vi "Functional Imaging Viewer.vi"(8 "error in (no error)":errorcluster, 11 "Experiment data folder path":path) -> ()   [LabVIEW 2013]
uses:
  Typedefs/ROI selector array-ROI vis.ctl
  xcontrol/Interface VIs/Interface typedefs/Interface-ROI selection cluster.ctl
  Typedefs/ROI ID Enum.ctl
  xcontrol/XGrapher.xctl
  Typedefs/Group sel cluster.ctl
  Typedefs/ROI visibility mode.ctl
  Typedefs/Functional Imging UI Refs.ctl
  Typedefs/Groups array referecne.ctl
  SubVIs/ROI grouping window/Typedefs/ROI grp-process states enum.ctl
  Typedefs/Registered event names enum.ctl
  Globals/gl_Funct imaging UI.vi
  Global variables/gl_Functional Imaging-Global variables.vi
panel:
  out "#of selected groups":i32 caption="MiniScans selected" format="%.0f Miniscans selected"
  out "Index of POI clicked on":i16
  out "Image":T1(plugin-control)
  out "Doc Min":dbl
  out "Doc Max":dbl
  in  "Z-Plane Selector":i32(c297)=7 caption="Z-Plane"
  out "Index of group clicked on":i16
  in  "ROI vis. mode":T2
  in  "Max Z-Projection":bool
  in  "Channel":u16(ring)=1 items=["Red", "Green"]
  in  "Intensity Zoom":cluster{u16, u16}(slide)={0, 694} scale=0.0..4095.0
  in  "Index of miniscan point to visualise":i32=1 min=1 max=61 step=1 format="Point %.0f"
  in  "Waveform selector":u16(ring) items=["Cursor on ROI 1 (MiniScan)"]
  out "XGrapher":T7(xcontrol)
  in  "Deselect all groups":bool=TRUE
  in  "Deselect all ROI":bool=TRUE
  out "Group info":string="0 of 0 groups selected"
  in  "[Groups]":T8[](array[typedef]) caption="Groups"
  out "Miniscan info":string="0 of 0 miniscans selected"
  out "POI info":string="0 of 0 POI selected"
  in  "Trial No.":i32=1 caption="Selected Trial" min=1 max=2 format="Trial %.0f"
  out "Number of Trials (ind1)":u16 min=1 max=16 format="of %.0d"
  in  "Smoothing":i32(slide) scale=0.0..10.0
  out "Number of Trials (ind 2)":u16 caption="Number of trials"
  out "Total # of points":i32 caption="Total number\nof loaded points"
  out "POI data points in each trial":i32
  out "#of selected POI":i32 caption="POI selected" format="%.0f POI selected"
  out "POI available":i32 caption="POI Available" format="%.0f POI available"
  out "MiniScans Available":i32 format="%.0f Miniscans available"
  out "#of selected MiniScans":i32 caption="MiniScans selected" format="%.0f Miniscans selected"
  in  "Defer graph updates":bool caption="Defer graph updates\non cursor move"
  in  "[ROI vis]":T9 caption="ROIs" {"ROI number" min=1 max=4 format="ROI %.0f"}
  in  "Show All":bool
  in  "Normalize":bool
  in  "POI Averaging":bool
  in  "Trial Cursor Enabled":bool caption="Trial Tracking Cursors"
  # "Cursors Settings"
  # "Post Processing Settings"
  # "Information"
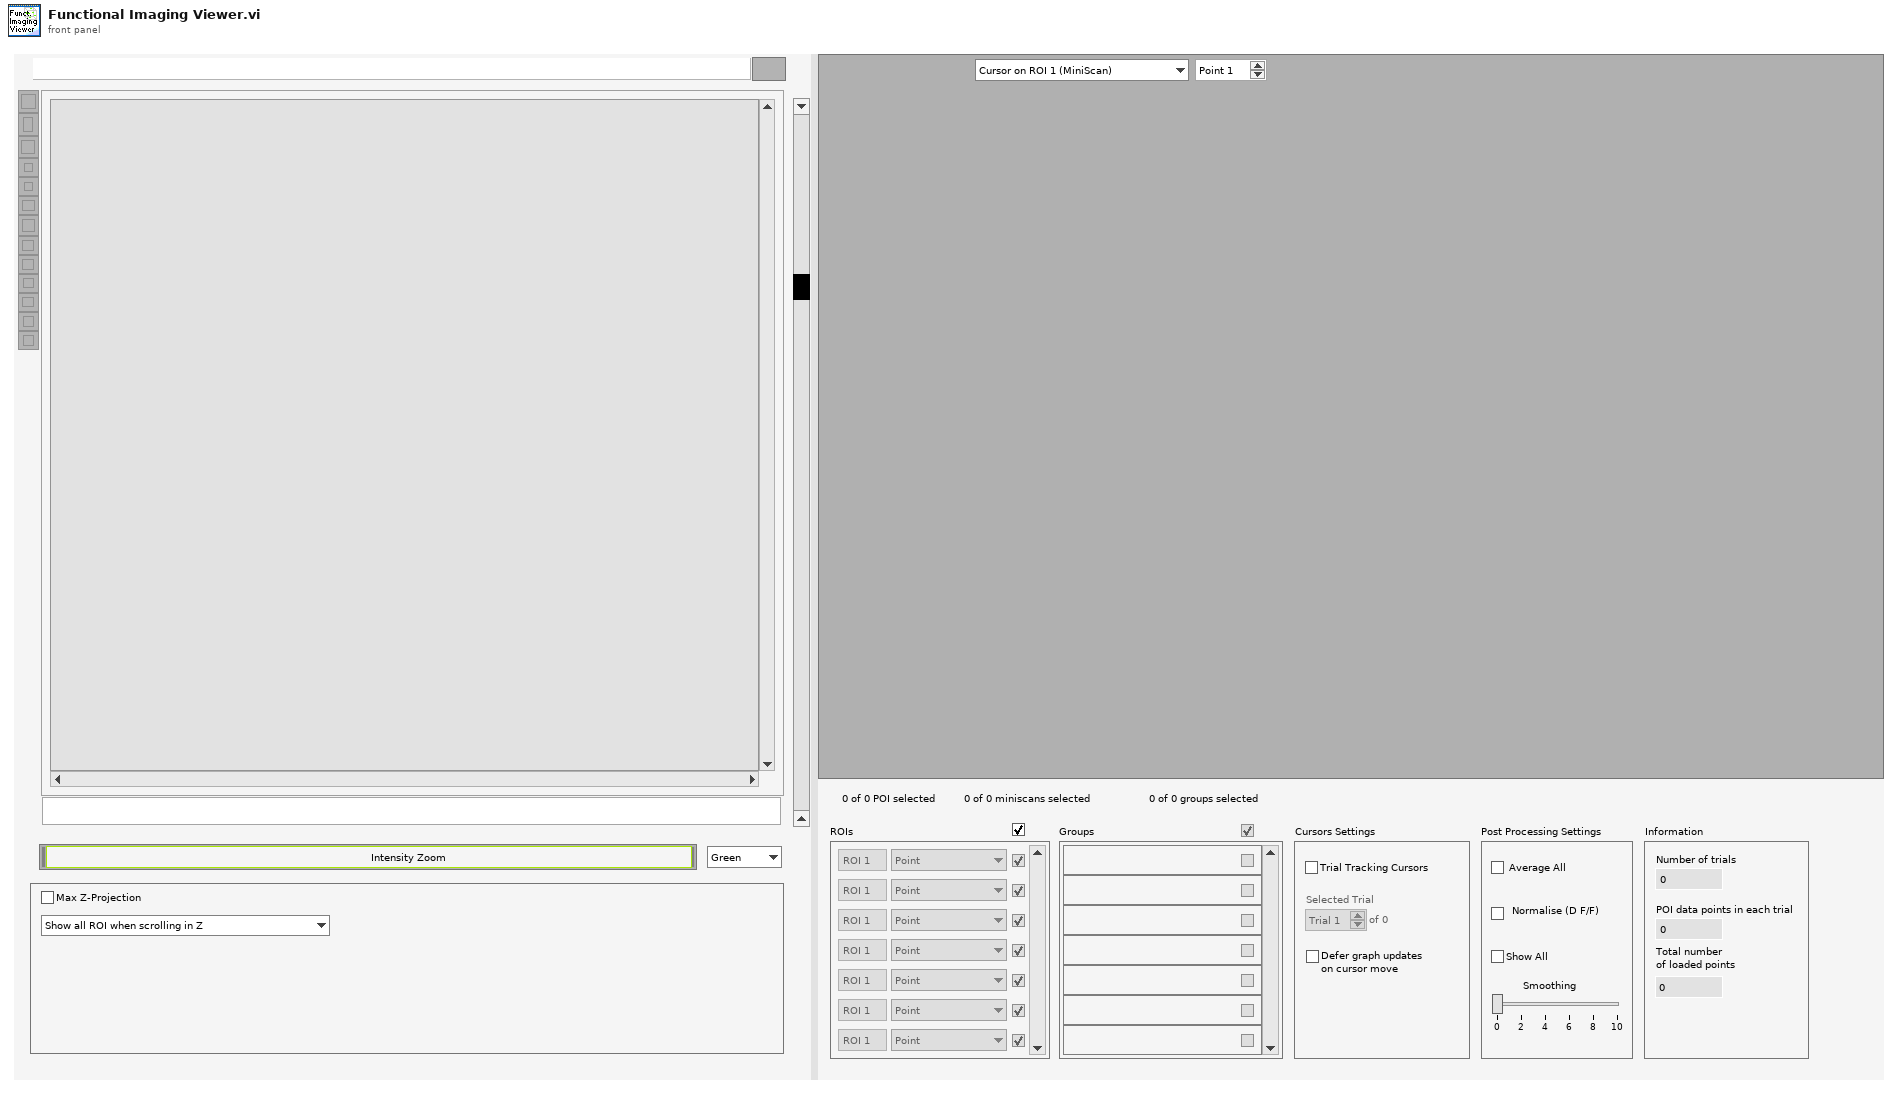
[diagram p1: front panel]
types:
  T1 = typedef "IMAQ Image.ctl" = refnum<image>
  T2 = typedef "ROI visibility mode.ctl" = enum16{"Show all ROI when scrolling in Z", "Show only selected ROI when scrolling in Z"}
  T3 = typedef "Xctrl-Data array.ctl" = T4[]
  T4 = typedef "XGrapher.xctl/Xcrtl-Data format definition.ctl" = cluster{"Plot.Plot Name":string, "Data":T5, "Timeline data":T5, "Type":T6, "Points per cycle":u16, "ROI index":u16}
  T5 = typedef "XGrapher.xctl/Xctl-XY data type definition.ctl" = cluster{"X-Axis values":sgl[], "Y-Axis values (s)":i32[]}
  T6 = typedef "Xctrl-ROI type enum.ctl" = enum16{"POI", "Mini-scan", "Group"}
  T7 = cluster{"Data & info by ROI index":T3, "Index of selected plot":u16, "Points in each trial":i32, "POI Averaging":bool, "Reset graph X-axis scaling":bool, "Selected point index in MSCN (unity based)":u16}
  T8 = typedef "Group sel cluster.ctl" = cluster{"Group number":string, "Group Name":string, "Visibility":bool, "Highlight":bool}
  T9 = typedef "ROI selector array-ROI vis.ctl" = T10[]
  T10 = typedef "Interface-ROI selection cluster.ctl" = cluster{"ROI number":i32, "ROI ID":T11, "Visibility":bool}
  T11 = typedef "ROI ID Enum.ctl" = enum16{"Point", "MiniScan", "Comp. MiniScan", "Rectangle", "Comp. volume", "Arb. plane point"}
  T12 = typedef "Functional Imging UI Refs.ctl" = cluster{"Menu ref":refnum<k9>, "Image control":refnum<vi>, "VI ref":refnum<vi>, "XGrapher":refnum<vi>, "Smoothing":refnum<vi>, "POI Averaging":refnum<vi>, "Normalize":refnum<vi>, "POI data points in each trial":refnum<vi>, "Channel":refnum<vi>, "Experiment data folder path":refnum<vi>, "[ROI vis]":refnum<vi>, "[Groups] visbl":T13, "Group Name":refnum<vi>, "POI index":refnum<vi>, "Trial No.":refnum<vi>, "Intensity Zoom":refnum<vi>, "Trial Cursor Enabled":refnum<vi>, "Number of Trials (ind 1)":refnum<vi>, "Number of Trials (ind 2)":refnum<vi>, "MiniScans Available":refnum<vi>, "POI Available":refnum<vi>, "Defer graph updates":refnum<vi>, "Waveform selector":refnum<vi>, "#of selected POI":refnum<vi>, "#of selected MiniScans":refnum<vi>, "#of selected groups":refnum<vi>, "Max Z-Projection":refnum<vi>, "Z-Plane Selector":refnum<vi>, "Index of miniscan point to visualise":refnum<vi>, "ROI vis. mode":refnum<vi>, "Total # of points":refnum<vi>, "Index of group clicked on":refnum<vi>, "Pane 1":refnum<vi>, "Pane 2":refnum<vi>, "Pane 3":refnum<vi>, "Pane 4":refnum<vi>, "Pane 5":refnum<vi>, "Pane 6":refnum<vi>, "Deselect all ROI":refnum<vi>, "Deselect all groups":refnum<vi>}
  T13 = typedef "Groups array referecne.ctl" = refnum<vi>
  T14 = typedef "Registered event names enum.ctl" = enum16{"Register", "Load dataset in funct viewer", "Re-process data", "Export selected ROI data-full"}
  T15 = typedef "ROI grp-process states enum.ctl" = enum16{"Open window", "Stop loop"}
  T16 = typedef "FuncImg-Events registration ref.ctl" = refnum<event-registration>
  T17 = typedef "eventsource.ctl" = u32
  T18 = typedef "Interface-ROI type enum.ctl" = enum16{"POI", "Mini-scan"}
  T19 = typedef "LVPoint32TypeDef.ctl" = cluster{"Horizontal":i32, "Vertical":i32}
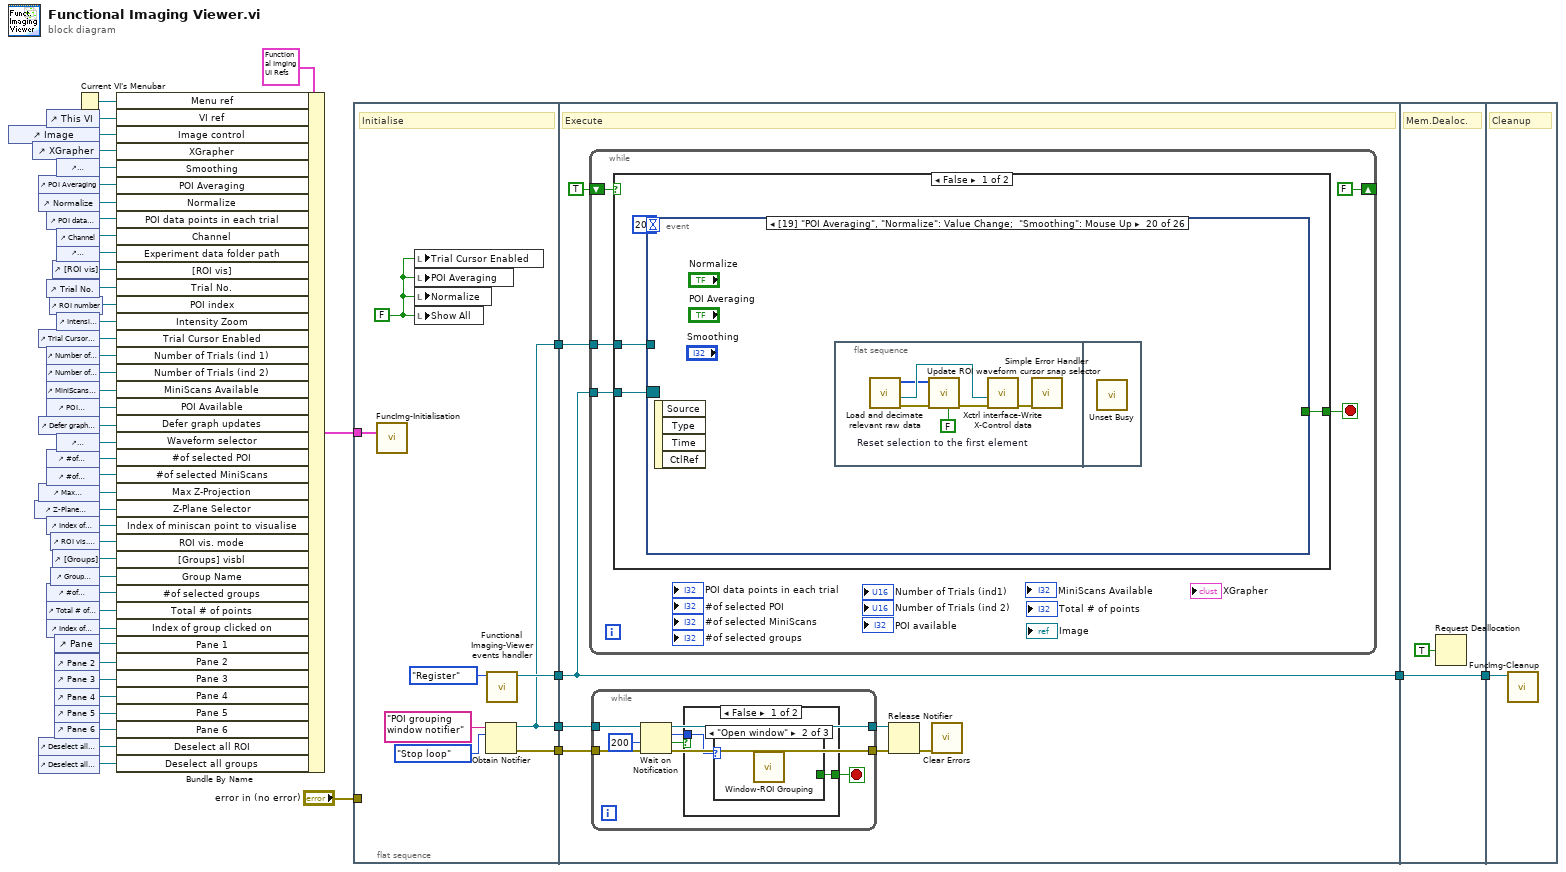
[diagram p0: block diagram]
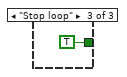
[diagram p3: hidden frame]
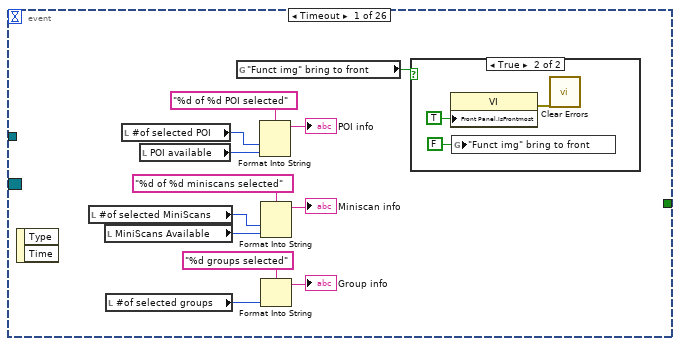
[diagram p5: hidden frame]
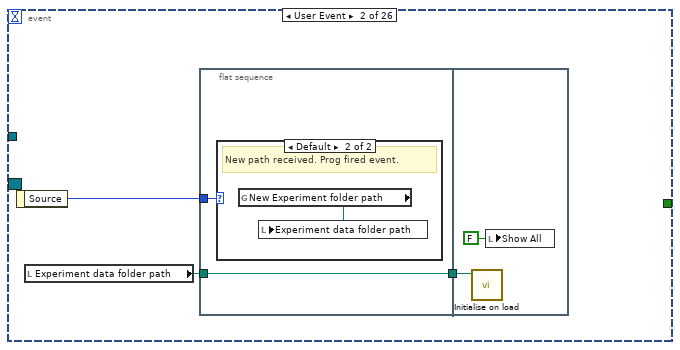
[diagram p7: hidden frame]
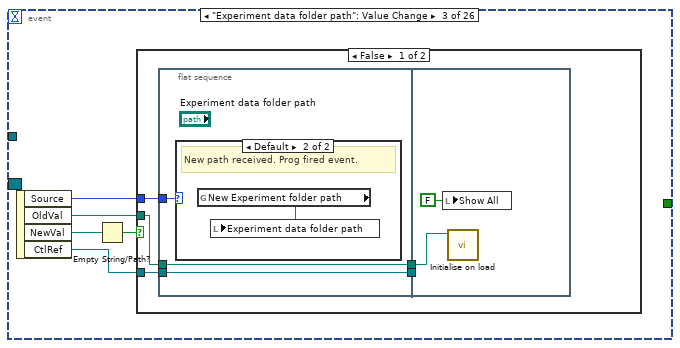
[diagram p9: hidden frame]
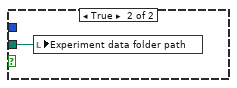
[diagram p11: hidden frame]
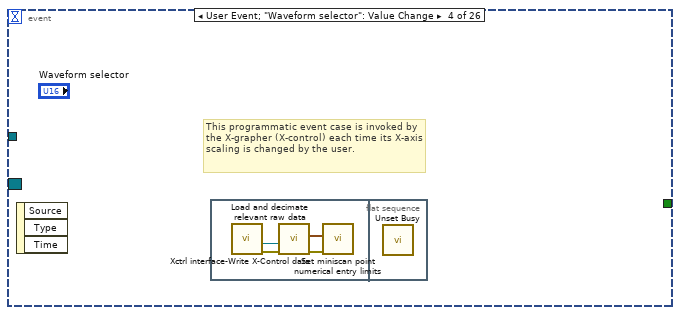
[diagram p12: hidden frame]
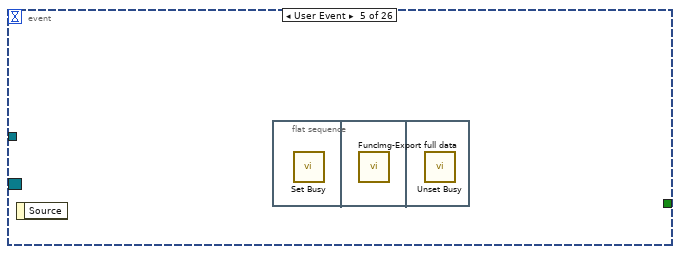
[diagram p13: hidden frame]
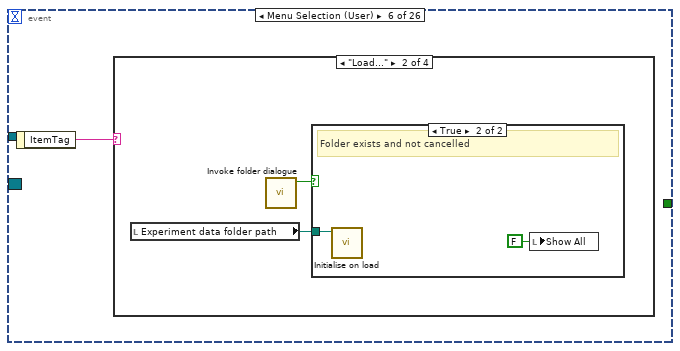
[diagram p14: hidden frame]
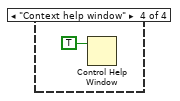
[diagram p18: hidden frame]
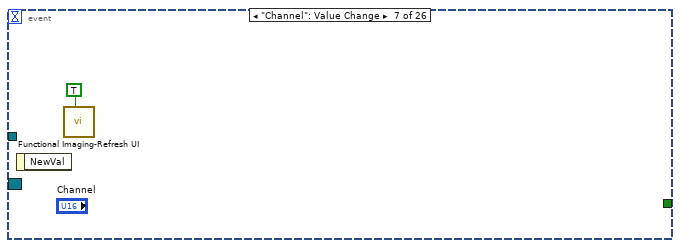
[diagram p19: hidden frame]
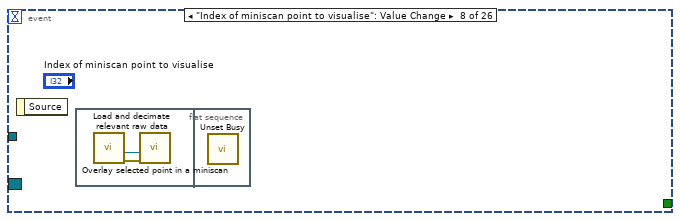
[diagram p20: hidden frame]
diagram:
  n1 = control-ref of="Image"() -> (w20:refnum<vi>)
  n2 = control-ref of="XGrapher"() -> (w32:refnum<vi>)
  n3 = control-ref of="Z-Plane Selector"() -> (w33:refnum<vi>)
  n4 = control-ref of="POI Averaging"() -> (w47:refnum<vi>)
  n5 = control-ref of="Normalize"() -> (w46:refnum<vi>)
  n6 = control-ref of="Trial Cursor Enabled"() -> (w41:refnum<vi>)
  n7 = control-ref of="Defer graph updates"() -> (w39:refnum<vi>)
  n8 = control-ref of="Max Z-Projection"() -> (w34:refnum<vi>)
  n9 = control-ref of="Deselect all ROI"() -> (w2:refnum<vi>)
  n10 = control-ref of="Deselect all groups"() -> (w1:refnum<vi>)
  n11 = control-ref of="This VI"() -> (w17:refnum<vi>)
  n12 = control-ref of="POI data points in each trial"() -> (w49:refnum<vi>)
  n13 = control-ref of="Trial No."() -> (w43:refnum<vi>)
  n14 = control-ref of="Number of Trials (ind1)"() -> (w40:refnum<vi>)
  n15 = control-ref of="Number of Trials (ind 2)"() -> (w29:refnum<vi>)
  n16 = control-ref of="MiniScans Available"() -> (w27:refnum<vi>)
  n17 = control-ref of="POI available"() -> (w28:refnum<vi>)
  n18 = control-ref of="#of selected POI"() -> (w36:refnum<vi>)
  n19 = control-ref of="#of selected MiniScans"() -> (w35:refnum<vi>)
  n20 = control-ref of="Index of miniscan point to visualise"() -> (w31:refnum<vi>)
  n21 = control-ref of="#of selected groups"() -> (w25:refnum<vi>)
  n22 = control-ref of="Total # of points"() -> (w19:refnum<vi>)
  n23 = control-ref of="Index of group clicked on"() -> (w18:refnum<vi>)
  n24 = control-ref of="ROI number"() -> (w37:refnum<vi>)
  n25 = control-ref of="ROI vis. mode"() -> (w26:refnum<vi>)
  n26 = control-ref of="Group Name"() -> (w3:refnum<vi>)
  n27 = control-ref of="[ROI vis]"() -> (w22:refnum<vi>)
  n28 = control-ref of="[Groups]"() -> (w21:refnum<vi>)
  n29 = control-ref of="Pane"() -> (w14:refnum<vi>)
  n30 = control-ref of="Pane 2"() -> (w13:refnum<vi>)
  n31 = control-ref of="Pane 3"() -> (w12:refnum<vi>)
  n32 = control-ref of="Pane 4"() -> (w11:refnum<vi>)
  n33 = control-ref of="Pane 5"() -> (w10:refnum<vi>)
  n34 = control-ref of="Pane 6"() -> (w9:refnum<vi>)
  n35 = control-ref of="Smoothing"() -> (w48:refnum<vi>)
  n36 = control-ref of="Channel"() -> (w45:refnum<vi>)
  n37 = control-ref of="Experiment data folder path"() -> (w44:refnum<vi>)
  n38 = control-ref of="Intensity Zoom"() -> (w42:refnum<vi>)
  n39 = control-ref of="Waveform selector"() -> (w38:refnum<vi>)
  n40 = Current VI's Menubar() -> (w4:refnum<k9>)
  n41 = Bundle By Name(cluster=T12 {"Menu ref"=refnum, "Image control"=refnum, "VI ref"=refnum, "XGrapher"=refnum, "Smoothing"=refnum, "POI Averaging"=refnum, "Normalize"=refnum, "POI data points in each trial"=refnum, "Channel"=refnum, "Experiment data folder path"=refnum, "[ROI vis]"=refnum, "[Groups] visbl"=refnum, "Group Name"=refnum, "POI index"=refnum, "Trial No."=refnum, "Intensity Zoom"=refnum, "Trial Cursor Enabled"=refnum, "Number of Trials (ind 1)"=refnum, "Number of Trials (ind 2)"=refnum, "MiniScans Available"=refnum, "POI Available"=refnum, "Defer graph updates"=refnum, "Waveform selector"=refnum, "#of selected POI"=refnum, "#of selected MiniScans"=refnum, "#of selected groups"=refnum, "Max Z-Projection"=refnum, "Z-Plane Selector"=refnum, "Index of miniscan point to visualise"=refnum, "ROI vis. mode"=refnum, "Total # of points"=refnum, "Index of group clicked on"=refnum, "Pane 1"=refnum, "Pane 2"=refnum, "Pane 3"=refnum, "Pane 4"=refnum, "Pane 5"=refnum, "Pane 6"=refnum, "Deselect all ROI"=refnum, "Deselect all groups"=refnum} ("Functional Imging UI Refs"), "Menu ref"=w4, "VI ref"=w17, "Image control"=w20, "XGrapher"=w32, "Smoothing"=w48, "POI Averaging"=w47, "Normalize"=w46, "POI data points in each trial"=w49, "Channel"=w45, "Experiment data folder path"=w44, "[ROI vis]"=w22, "Trial No."=w43, "POI index"=w37, "Intensity Zoom"=w42, "Trial Cursor Enabled"=w41, "Number of Trials (ind 1)"=w40, "Number of Trials (ind 2)"=w29, "MiniScans Available"=w27, "POI Available"=w28, "Defer graph updates"=w39, "Waveform selector"=w38, "#of selected POI"=w36, "#of selected MiniScans"=w35, "Max Z-Projection"=w34, "Z-Plane Selector"=w33, "Index of miniscan point to visualise"=w31, "ROI vis. mode"=w26, "[Groups] visbl"=w21, "Group Name"=w3, "#of selected groups"=w25, "Total # of points"=w19, "Index of group clicked on"=w18, "Pane 1"=w14, "Pane 2"=w13, "Pane 3"=w12, "Pane 4"=w11, "Pane 5"=w10, "Pane 6"=w9, "Deselect all ROI"=w2, "Deselect all groups"=w1) -> (w16:T12)
  n42 = flat-sequence {
    tunnel: w16 -> [w51]
    tunnel: "error in (no error)" -> [_]
    tunnel: [w56] -> w8
    tunnel: [w55] -> w7
    tunnel: [w54] -> w6
    tunnel: [w54] -> w5
    tunnel: w8 -> [w64]
    tunnel: [w64] -> w24
    tunnel: w7 -> [w63]
    tunnel: w6 -> [w62]
    tunnel: w5 -> [w60]
    tunnel: w24 -> [w178]
    tunnel: [w178] -> w15
    tunnel: w15 -> [w180]
    frame #0 {
      w57 = FALSE
      # "Initialise"
      n43 = call "FuncImg-Initialisation.vi"("Functional Imging UI Refs"=w51) -> ()  [unwired: 11 in]
      n44 = local write "Trial Cursor Enabled"(w57) -> ()
      n45 = local write "POI Averaging"(w57) -> ()
      n46 = local write "Normalize"(w57) -> ()
      n47 = local write "Show All"(w57) -> ()
      n48 = Obtain Notifier(name (unnamed)="POI grouping window notifier", notification data type=ROI_grp-process_states_enum."Stop loop" ("Function")) -> (notifier out=w54:refnum<notifier>, error out=w55:errorcluster)  [unwired: 2 in, 1 out]
      n49 = call "Functional Imaging-Viewer events handler.vi"("Event Function"=Registered_event_names_enum."Register") -> ("Event Registration Refnum"=w56:T16)  [unwired: 9 in, 1 out]
    }
    frame #1 {
      # "Execute"
      n50 = while {
        shift-right: [FALSE ("\"Funct img\" window is open")] -> _
        shift-left: TRUE ("\"Funct img\" window is open") -> [w80]
        tunnel: w64 -> [w78]
        tunnel: w60 -> [w77]
        stop <- w81 stop-if-true
        n51 = case shown="False" w80 {
          tunnel: [w85 _] -> w81
          tunnel: w78 -> [w83 _]
          tunnel: w77 -> [w82 _]
          frame False {
            n52 = event shown="[19] \"POI Averaging\", \"Normalize\": Value Change;  \"Smoothing\": Mouse Up" {
              selector: w83 -> [_ _ _ _ _ _ _ _ _ _ _ _ _ _ _ _ _ _ _ _ _ _ _ _ _ _]
              dyn-events: _ -> [_ _ _ _ _ _ _ _ _ _ _ _ _ _ _ _ _ _ _ _ _ _ _ _ _ _]
              timeout: 200 -> [_ _ _ _ _ _ _ _ _ _ _ _ _ _ _ _ _ _ _ _ _ _ _ _ _ _]
              tunnel: [_ _ _ _ _ _ _ _ _ _ _ _ _ _ _ _ _ _ _ _ _ _ w163 _ _ _] -> w85
              tunnel: w82 -> [_ _ _ _ _ _ _ _ _ _ _ _ _ _ _ _ _ w155 _ _ _ _ w164 _ _ _]
              event Timeout {
                n53 = event-data() -> ()  [unwired: 1 in, 2 out]
                n54 = local read "#of selected MiniScans"() -> (w88:i32)
                n55 = local read "MiniScans Available"() -> (w87:i32)
                n56 = local read "#of selected groups"() -> (w86:i32)
                n57 = local read "#of selected POI"() -> (w93:i32)
                n58 = local read "POI available"() -> (w92:i32)
                n59 = global read "gl_Funct imaging UI.vi" "\"Funct img\" bring to front"() -> (w97:bool)
                n60 = Format Into String(format string="%d of %d POI selected", w93, w92) -> (resulting string=→"POI info":string)  [unwired: 2 in, 1 out]
                n61 = Format Into String(format string="%d of %d miniscans selected", w88, w87) -> (resulting string=→"Miniscan info":string)  [unwired: 2 in, 1 out]
                n62 = Format Into String(format string="%d groups selected", w86) -> (resulting string=→"Group info":string)  [unwired: 2 in, 1 out]
                n63 = case shown="True" w97 {
                  frame False {
                  }
                  frame True {
                    n64 = property class="VI"("Front Panel.IsFrontmost"=TRUE ("Front Panel Window:Is Frontmost")) -> (error out=w99:errorcluster)  [unwired: 2 in, 1 out]
                    n65 = global write "gl_Funct imaging UI.vi" "\"Funct img\" bring to front"(FALSE ("\"Funct img\" bring to front")) -> ()
                    n66 = call <vilib>:"Clear Errors.vi"("error in (no error)"=w99) -> ()  [unwired: 6 in, 1 out]
                  }
                }
              }
              event User Event {
                n67 = event-data() -> ("Source"=w103:T17)  [unwired: 1 in]
                n68 = local read "Experiment data folder path"() -> (w101:path)
                n69 = flat-sequence {
                  tunnel: w103 -> [w105]
                  tunnel: [w104] -> w102
                  tunnel: w101 -> [w104]
                  tunnel: w102 -> [w107]
                  frame #0 {
                    n70 = case shown="Default" w105 {
                      frame 0 {
                        # "Path changed directly by the user"
                      }
                      frame Default {
                        # "New path received. Prog fired event."
                        n71 = global read "gl_Funct imaging UI.vi" "New Experiment folder path"() -> (w106:path)
                        n72 = local write "Experiment data folder path"(w106) -> ()
                      }
                    }
                  }
                  frame #1 {
                    n73 = call "Initialise on load.vi"("OldVal"=w107) -> ()  [unwired: 11 in]
                    n74 = local write "Show All"(FALSE ("Show All")) -> ()
                  }
                }
              }
              event "Experiment data folder path": Value Change {
                n75 = event-data() -> ("Source"=w113:T17, "OldVal"=w110:path, "NewVal"=w112:path, "CtlRef"=w109:refnum<vi>)  [unwired: 1 in]
                n76 = Empty String/Path?(string/path=w112) -> (empty?=w111:bool)
                n77 = case shown="False" w111 {
                  tunnel: w113 -> [w118 _]
                  tunnel: w110 -> [w114 w125]
                  tunnel: w109 -> [w116 _]
                  frame False {
                    n78 = flat-sequence {
                      tunnel: w118 -> [w121]
                      tunnel: [w120] -> w117
                      tunnel: w116 -> [w120]
                      tunnel: [w119] -> w115
                      tunnel: w114 -> [w119]
                      tunnel: w117 -> [_]
                      tunnel: w115 -> [w123]
                      frame #0 {
                        n79 = case shown="Default" w121 {
                          frame 0 {
                            # "Path changed directly by the user"
                          }
                          frame Default {
                            # "New path received. Prog fired event."
                            n80 = global read "gl_Funct imaging UI.vi" "New Experiment folder path"() -> (w122:path)
                            n81 = local write "Experiment data folder path"(w122) -> ()
                          }
                        }
                      }
                      frame #1 {
                        n82 = local write "Show All"(FALSE ("Show All")) -> ()
                        n83 = call "Initialise on load.vi"("OldVal"=w123) -> ()  [unwired: 11 in]
                      }
                    }
                  }
                  frame True {
                    n84 = local write "Experiment data folder path"(w125) -> ()
                  }
                }
              }
              event User Event; "Waveform selector": Value Change {
                # "This programmatic event case is invoked by the X-grapher (X-control) each time its X-axis scaling is changed by the user."
                n85 = event-data() -> ()  [unwired: 1 in, 3 out]
                n86 = flat-sequence {
                  frame #0 {
                    n87 = call "Load and decimate relevant raw data.vi"() -> ("error out"=w127:errorcluster, "Data reference"=w128:refnum<data-value>)  [unwired: 7 in, 3 out]
                    n88 = call "Xctrl interface-Write X-Control data.vi"("error in (no error)"=w127, "Data reference"=w128) -> ("error out"=w126:errorcluster, "Properties of selected ROI"=w129:cluster{"Type":T18, "Points per cycle":u16})  [unwired: 8 in]
                    n89 = call "Set miniscan point numerical entry limits.vi"("error in"=w126, "Properties of selected ROI"=w129) -> ()  [unwired: 9 in, 1 out]
                  }
                  frame #1 {
                    n90 = call <vilib>:"Unset Busy.vi"() -> ()  [unwired: 11 in, 1 out]
                  }
                }
              }
              event User Event {
                n91 = event-data() -> ()  [unwired: 1 in, 1 out]
                n92 = flat-sequence {
                  frame #0 {
                    n93 = call <vilib>:"Set Busy.vi"() -> ()  [unwired: 10 in, 2 out]
                  }
                  frame #1 {
                    n94 = call "FuncImg-Export full data.vi"() -> ()  [unwired: 10 in, 2 out]
                  }
                  frame #2 {
                    n95 = call <vilib>:"Unset Busy.vi"() -> ()  [unwired: 11 in, 1 out]
                  }
                }
              }
              event Menu Selection (User) {
                n96 = event-data() -> ("ItemTag"=w130:string)  [unwired: 1 in]
                n97 = case shown="\"Load...\"" w130 {
                  frame Default {
                  }
                  frame "Load..." {
                    n98 = local read "Experiment data folder path"() -> (w131:path)
                    n99 = call "Invoke folder dialogue.vi"() -> ("Folder exists & not cancelled"=w132:bool)  [unwired: 10 in, 1 out]
                    n100 = case shown="True" w132 {
                      tunnel: w131 -> [_ w133]
                      frame False {
                        # "Folder not found OR user cancelled"
                      }
                      frame True {
                        # "Folder exists and not cancelled"
                        n101 = call "Initialise on load.vi"("OldVal"=w133) -> ()  [unwired: 11 in]
                        n102 = local write "Show All"(FALSE ("Show All")) -> ()
                      }
                    }
                  }
                  frame "Export..." {
                  }
                  frame "Context help window" {
                    n103 = Control Help Window(1:TRUE ("Show")) -> ()  [unwired: 1 in]
                  }
                }
              }
              event "Channel": Value Change {
                n104 = event-data() -> ()  [unwired: 1 in, 1 out]
                n105 = call "Functional Imaging-Refresh UI.vi"("Reset graph X-axis scaling (F)"=TRUE) -> ()  [unwired: 11 in]
              }
              event "Index of miniscan point to visualise": Value Change {
                n106 = event-data() -> ()  [unwired: 1 in, 1 out]
                n107 = flat-sequence {
                  frame #0 {
                    n108 = call "Load and decimate relevant raw data.vi"() -> ("error out"=w138:errorcluster, "Data reference"=w137:refnum<data-value>)  [unwired: 7 in, 3 out]
                    n109 = call "Overlay selected point in a miniscan.vi"("error in"=w138, "Data reference"=w137) -> ()  [unwired: 9 in, 1 out]
                  }
                  frame #1 {
                    n110 = call <vilib>:"Unset Busy.vi"() -> ()  [unwired: 11 in, 1 out]
                  }
                }
              }
              event Value Change {
                n111 = event-data() -> ("OldVal"=w139:T9, "NewVal"=w140:T9)  [unwired: 1 in]
                n112 = call "FuncImg-Event handler-ROI visibl value change.vi"("NewVal"=w140, "OldVal"=w139) -> ()  [unwired: 10 in]
              }
              event Shortcut Menu Activation? {
                n113 = event-data() -> ("CtlRef"=w141:refnum<vi>, "Coords"=w143:T19)  [unwired: 1 in]
                n114 = call "Coords_to_Index.vi"("coords"=w143, "Array ref"=w141) -> ("row index"=→"Index of POI clicked on":i16)  [unwired: 5 in, 4 out]
                n115 = event-data() -> ()  [unwired: 2 in, 1 out]
              }
              event "Deselect all ROI": Value Change {
                n116 = event-data() -> ("NewVal"=w144:bool)  [unwired: 1 in]
                n117 = call "Deselect All ROI.vi"("Deselect all ROI"=w144) -> ()  [unwired: 10 in, 1 out]
              }
              event "Deselect all groups": Value Change {
                n118 = event-data() -> ("NewVal"=w145:bool)  [unwired: 1 in]
                n119 = call "Deselect All groups.vi"("Deselect all groups"=w145) -> ()  [unwired: 10 in, 1 out]
              }
              event "[Groups]": Value Change {
                n120 = event-data() -> ("CtlRef"=w146:refnum<vi>, "NewVal"=w147:T8[], "OldVal"=w148:T8[])  [unwired: 1 in]
                n121 = call "ROI group-Event handler-Groups array value change.vi"("OldVal"=w148, "NewVal"=w147, "[Groups]"=w146) -> ()  [unwired: 9 in]
              }
              event "[Groups]": Mouse Move {
                n122 = event-data() -> ("CtlRef"=w150:refnum<vi>, "Coords"=w149:T19)  [unwired: 1 in]
                n123 = call "ROI group-Event handler-ROI group mouse move.vi"("Coords"=w149, "[Groups]"=w150) -> ()  [unwired: 9 in, 1 out]
              }
              event "[Groups]": Mouse Down {
                n124 = event-data() -> ("Coords"=w151:T19)  [unwired: 1 in]
                n125 = call "Validate and register ROI group clicked on.vi"("Coords"=w151) -> ()  [unwired: 8 in, 3 out]
              }
              event "[Groups]": Mouse Up {
                n126 = event-data() -> ("Coords"=w152:T19)  [unwired: 1 in]
                n127 = call "FuncImg-Event handler-Groups mouse up.vi"("Coords"=w152) -> ()  [unwired: 11 in]
              }
              event "[Groups]": Shortcut Menu Activation? {
                n128 = event-data() -> ("MenuRef"=w153:refnum<k9>, "Coords"=w154:T19)  [unwired: 1 in]
                n129 = call "ROI group-Event handler-Shortcut menu activ.vi"("Coords"=w154, "[Groups] menu ref"=w153) -> ()  [unwired: 9 in, 1 out]
                n130 = event-data() -> ()  [unwired: 2 in, 1 out]
              }
              event "[Groups]": Shortcut Menu Selection (User) {
                n131 = event-data() -> ("ItemTag"=w156:string)  [unwired: 1 in]
                n132 = call "ROI group-Groups control menu handler.vi"("ItemTag"=w156, "ROI groups window notifier"=w155) -> ()  [unwired: 10 in]
              }
              event "Intensity Zoom": Value Change {
                # "Rescale Image display's Z-axis"
                n133 = event-data() -> ()  [unwired: 1 in, 1 out]
                n134 = call "Functional Imaging-16bit display mapping.vi"() -> ()  [unwired: 11 in, 1 out]
              }
              event "POI Averaging", "Normalize": Value Change; "Smoothing": Mouse Up {
                n135 = event-data() -> ()  [unwired: 1 in, 4 out]
                n136 = flat-sequence {
                  frame #0 {
                    w159 = FALSE  # Reset selection to the first element
                    n137 = call "Load and decimate relevant raw data.vi"() -> ("error out"=w160:errorcluster, "Data reference"=w162:refnum<data-value>, "Sorted Pointers"=w161:i32[])  [unwired: 7 in, 2 out]
                    n138 = call "Update ROI waveform cursor snap selector.vi"("Reset selection to the first element"=w159, "error in (no error)"=w160, "Sorted Pointers"=w161) -> ("error out"=w158:errorcluster)  [unwired: 8 in]
                    n139 = call "Xctrl interface-Write X-Control data.vi"("error in (no error)"=w158, "Data reference"=w162) -> ("error out"=w157:errorcluster)  [unwired: 8 in, 1 out]
                    n140 = call <vilib>:"Simple Error Handler.vi"("error in (no error)"=w157) -> ()  [unwired: 4 in, 5 out]
                  }
                  frame #1 {
                    n141 = call <vilib>:"Unset Busy.vi"() -> ()  [unwired: 11 in, 1 out]
                  }
                }
              }
              event "Show All": Value Change {
                n142 = event-data() -> ()  [unwired: 1 in, 1 out]
                n143 = call "FuncImg-Show all ROI.vi"() -> ()  [unwired: 11 in, 1 out]
              }
              event "Defer graph updates": Value Change {
                n144 = event-data() -> ()  [unwired: 1 in, 1 out]
                n145 = call "Xctrl interface-Defer graph updates.vi"() -> ()  [unwired: 11 in, 1 out]
              }
              event Panel Close? {
                n146 = event-data() -> ()  [unwired: 1 in, 1 out]
                n147 = call "Dialogue Window.vi"("Caption-Left button (Cancel)"="Cancel" ("F button name (\"Cancel\")"), "Caption-Right button (OK)"="Close" ("T button name (\"OK\")"), "Message string"="Are you sure you want to close the functional imaging viewer?" ("message")) -> ("Cancelled (Left button pressed)"=w168:bool)  [unwired: 6 in, 2 out]
                n148 = Not(x=w168) -> (.not. x?=w163:bool)
                n149 = case shown="True" w163 {
                  tunnel: w164 -> [_ w172]
                  frame False {
                  }
                  frame True {
                    n150 = global write "gl_Functional Imaging-Global variables.vi" "Functional viewer closing"(TRUE ("Functional viewer closing")) -> ()
                    n151 = Send Notification(notification=ROI_grp-process_states_enum."Stop loop" ("Function"), notifier=w172) -> ()  [unwired: 1 in, 2 out]
                  }
                }
                n152 = event-data("Discard?"=TRUE) -> ()  [unwired: 1 in, 1 out]
              }
              event "Trial Cursor Enabled", "Trial No.": Value Change {
                n153 = event-data() -> ()  [unwired: 1 in, 1 out]
                n154 = call "Xctrl interface-Set trial cursors.vi"() -> ()  [unwired: 11 in, 1 out]
                n155 = call "Functional Imaging-Trial number disabled state.vi"() -> ()  [unwired: 12 in]
              }
              event "Max Z-Projection": Value Change {
                n156 = event-data() -> ()  [unwired: 1 in, 1 out]
                n157 = call "Functional Imaging-Add Z-stack images handler.vi"() -> ()  [unwired: 11 in, 1 out]
              }
              event "Z-Plane Selector": Value Change {
                # "Debugging controls.\nNormally hidden."
                n158 = event-data() -> ()  [unwired: 1 in, 1 out]
                n159 = call "FuncImg-Event handler-Z plane value change.vi"() -> ()  [unwired: 12 in]
                n160 = call "Get Z selector Doc max min.vi"() -> ("DocMin"=→"Doc Min":dbl, "DocMax"=→"Doc Max":dbl)  [unwired: 10 in]
              }
            }
          }
          frame True {
            n161 = flat-sequence {
              frame #0 {
                n162 = local read "Experiment data folder path"() -> (w175:path)
                n163 = local write "Show All"(FALSE ("Show All")) -> ()
                n164 = call "Initialise on load.vi"("OldVal"=w175) -> ()  [unwired: 11 in]
              }
              frame #1 {
                # "Set true after initialisation is complete"
                n165 = global write "gl_Funct imaging UI.vi" "\"Funct img\" window is open"(TRUE ("\"Funct img\" window is open")) -> ()
              }
            }
          }
        }
      }
      n166 = while {
        tunnel: w63 -> [w73]
        tunnel: w62 -> [w72]
        tunnel: [w70] -> w61
        tunnel: [w66] -> w58
        stop <- w67 stop-if-true
        n167 = Wait on Notification(notifier=w72, timeout in ms (-1)=200, error in (no error)=w73) -> (notifier out=w70:refnum<notifier>, notification=w68:T15, timed out?=w69:bool, error out=w66:errorcluster)  [unwired: 1 in]
        n168 = case shown="False" w69 {
          tunnel: w68 -> [w75 _]
          tunnel: [w74 _] -> w67
          frame False {
            n169 = case shown="\"Open window\"" w75 {
              tunnel: [_ _ TRUE] -> w74
              frame Default {
              }
              frame "Open window" {
                n170 = call "Window-ROI Grouping.vi"() -> ()  [unwired: 12 in]
              }
              frame "Stop loop" {
              }
            }
          }
          frame True {
          }
        }
      }
      n171 = Release Notifier(notifier=w61, error in (no error)=w58) -> (error out=w59:errorcluster)  [unwired: 1 in, 2 out]
      n172 = call <vilib>:"Clear Errors.vi"("error in (no error)"=w59) -> ()  [unwired: 6 in, 1 out]
    }
    frame #2 {
      # "Mem.Dealoc."
      n173 = Request Deallocation(TRUE ("flag")) -> ()
    }
    frame #3 {
      # "Cleanup"
      n174 = call "FuncImg-Cleanup.vi"("Event Registration Refnum in"=w180) -> ()  [unwired: 11 in]
    }
  }
